vi "Config Key String To Numeric ID String Map.vi"(7 "Section In":string, 8 "Error In":errorcluster, 9 "ID In":i64[](array[numeric]), 10 "Keys In":string[](array[string]), 11 "Ref In":T1) -> (0 "Error Out":errorcluster, 2 "Numeric Map Out":map{i64, string}(c390), 3 "Ref Out":T1)   [LabVIEW 2024]
uses:
  <vilib>/Utility/config.llb/Config Data RefNum.ctl
  <vilib>/Utility/config.llb/Read Key (String).vi
  <vilib>/Utility/config.llb/NI_LVConfig.lvlib
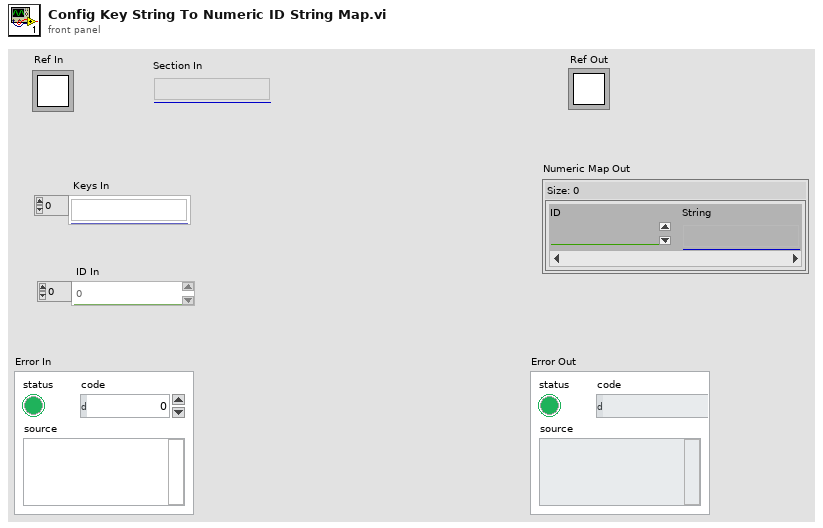
[diagram p1: front panel]
types:
  T1 = typedef "NI_LVConfig.lvlib/Config Data RefNum.ctl" = refnum<k1>
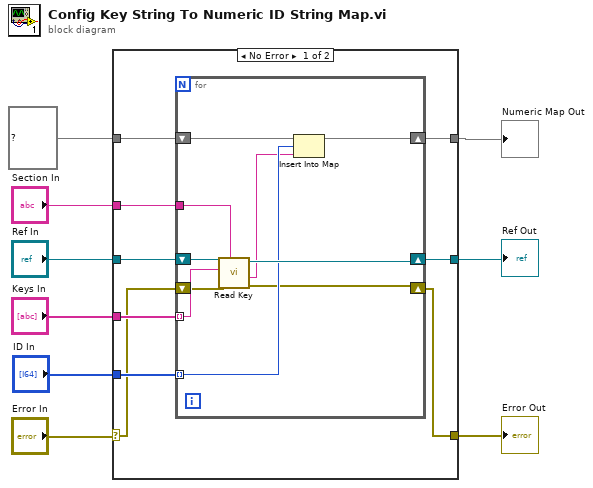
[diagram p0: block diagram]
diagram:
  n1 = case shown="No Error" "Error In" {
    selector: "Error In" -> [w12 w30]
    tunnel: "Ref In" -> [w18 w31]
    tunnel: [w17 w31] -> w8
    tunnel: "Section In" -> [w16 _]
    tunnel: [w10 w30] -> w5
    tunnel: "Keys In" -> [w15 _]
    tunnel: "ID In" -> [w14 _]
    tunnel: map{i64, string} {} ("Numeric Map Out") -> [w13 w29]
    tunnel: [w11 w29] -> w1
    frame No Error {
      n2 = for {
        shift-right: [w26] -> w17
        shift-left: w18 -> [w28]
        tunnel: w16 -> [w27]
        tunnel: w15 -> [w25] mode=indexing
        tunnel: w14 -> [w23] mode=indexing
        shift-right: [w19] -> w11
        shift-left: w13 -> [w24]
        shift-right: [w20] -> w10
        shift-left: w12 -> [w21]
        n3 = call-poly <vilib>:"Read Key.vi"("section"=w27, "error in (no error)"=w21, "key"=w25, "refnum"=w28) -> ("error out"=w20:errorcluster, "value"=w22:string, "refnum out"=w26:T1)  [unwired: 4 in, 1 out]
        n4 = Insert Into Map(map in=w24, key=w23, value=w22) -> (map out=w19:map{i64, string})  [unwired: 2 out]
      }
    }
    frame Error {
    }
  }
  "Ref Out" <- w8
  "Error Out" <- w5
  "Numeric Map Out" <- w1
